vi "runtest Print Selected Reports.vi"(0 "Fields":T1[](array[typedef])=[{"ixField"=0, "iSequenceOrder"=0, "sxFieldId"="Serial Number", "sxSequenceId"="", "sDisplayName"="test", "sValue"="", "sUnits"="", "nDataType"=enum."timestamp", "nNextItem"=enum."Reset", "fSystem"=FALSE, "fSystemValue"=FALSE, "fRequired"=FALSE, "fSetAtTest"=FALSE, "fTestField"=FALSE, "fDeleted"=FALSE, "fIndexed"=FALSE, "fFreeList"=FALSE}, {"ixField"=0, "iSequenceOrder"=0, "sxFieldId"="Model Number", "sxSequenceId"="", "sDisplayName"="test", "sValue"="", "sUnits"="", "nDataType"=enum."timestamp", "nNextItem"=enum."Reset", "fSystem"=FALSE, "fSystemValue"=FALSE, "fRequired"=FALSE, "fSetAtTest"=FALSE, "fTestField"=FALSE, "fDeleted"=FALSE, "fIndexed"=FALSE, "fFreeList"=FALSE}], 1 "sDatasheetsCSV (\"\")":string, 3 "sTestId":string, 5 "Data File Path":path, 9 "Run ID String (\"\")":string, 11 "error in (no error)":errorcluster, 12 "Test Station IP (\"\")":string, 13 "Save Results?":bool, 14 "sxUsername (\"\")":string) -> (15 "error out":errorcluster)   [LabVIEW 2011]
uses:
  server/database/Fields/Field Record.ctl
  server/database/Fields/Field DataTypes.ctl
  server/database/Fields/Field NextItem.ctl
  server/DIAdem/Datasheet/Datasheet Generator Settings.ctl
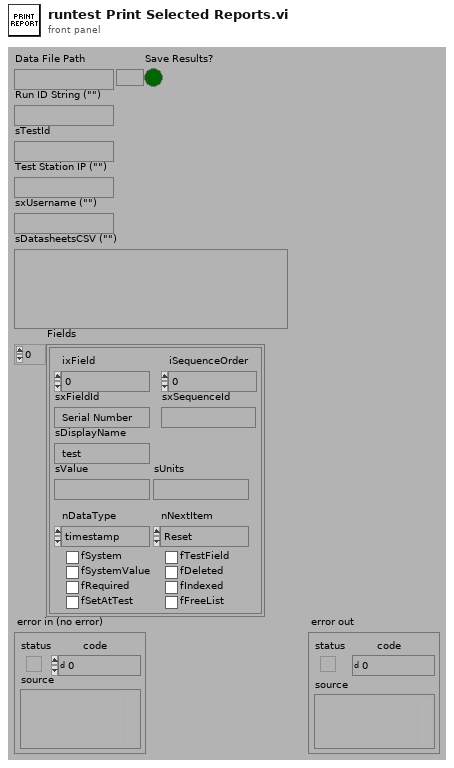
[diagram p1: front panel]
types:
  T1 = typedef "Field Record.ctl" = cluster{"ixField":i32, "iSequenceOrder":i32, "sxFieldId":string, "sxSequenceId":string, "sDisplayName":string, "sValue":string, "sUnits":string, "nDataType":T2, "nNextItem":T3, "fSystem":bool, "fSystemValue":bool, "fRequired":bool, "fSetAtTest":bool, "fTestField":bool, "fDeleted":bool, "fIndexed":bool, "fFreeList":bool}
  T2 = typedef "Field DataTypes.ctl" = enum32{"text", "numeric", "list", "timestamp", "boolean"}
  T3 = typedef "Field NextItem.ctl" = enum32{"Reset", "Retain", "Auto-Increment"}
  T4 = typedef "DATASHEET Generator Settings.ctl" = cluster{"Wait? (t)":bool, "ClientPrint? (f)":bool, "Client (\"\")":string, "joinPDF":bool, "Sort Method":enum16{"Item", "Template", "No Sort"}, "Export Row (-1=all)":i32, "Preview":bool, "Estimate Time":bool, "username":string, "jobid":string}
  T5 = typedef "Connection Refnum.ctl" = cluster{"Environment Handle":i32, "Connection Handle":i32}
  T6 = typedef "TDM_INDEX Record.ctl" = cluster{"Model Number":string, "SN for sort":i32, "Test Type":string, "Test Run":string, "Serial Number":string, "Start Timestamp":timestamp, "Data File":path, "Result Columns":string[]}
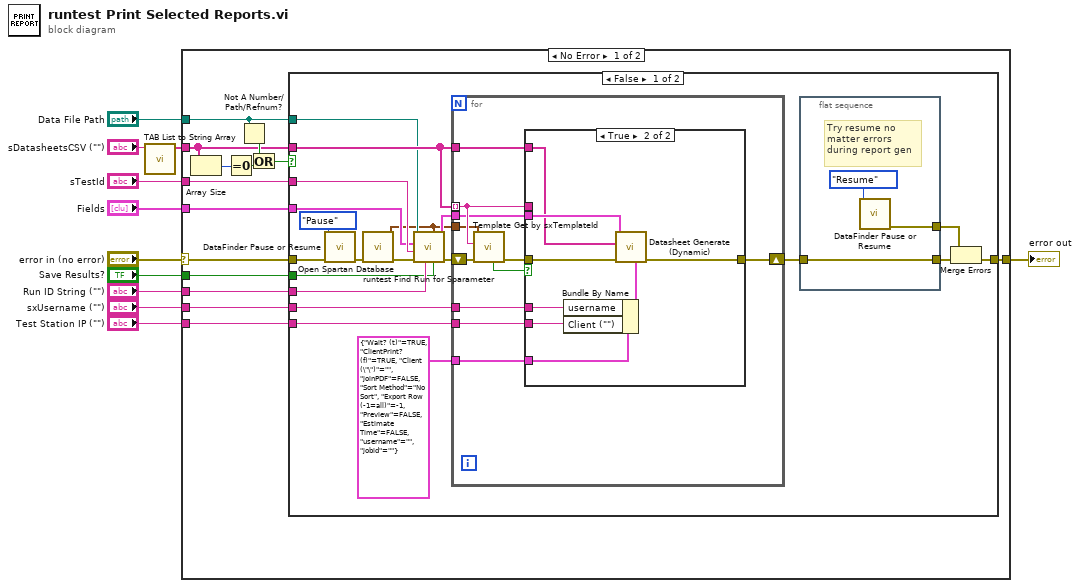
[diagram p0: block diagram]
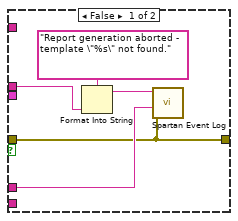
[diagram p2: hidden frame]
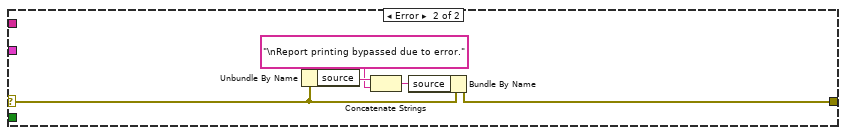
[diagram p4: hidden frame]
diagram:
  n1 = call "TAB List to String Array.vi"("String"="sDatasheetsCSV (\"\")") -> ("Array"=w3:string[])  [unwired: 10 out]
  n2 = case shown="No Error" "error in (no error)" {
    selector: "error in (no error)" -> [w18 w75]
    tunnel: [w21 w74] -> w11
    tunnel: "sxUsername (\"\")" -> [w19 _]
    tunnel: "Run ID String (\"\")" -> [w17 _]
    tunnel: "Data File Path" -> [w12 _]
    tunnel: w3 -> [w15 _]
    tunnel: "Test Station IP (\"\")" -> [w20 _]
    tunnel: "Fields" -> [w16 _]
    tunnel: "sTestId" -> [w14 _]
    tunnel: "Save Results?" -> [w13 _]
    frame No Error {
      n3 = Array Size(array=w15) -> (size(s)=w25:i32)
      n4 = Equal To 0?(x=w25) -> (x = 0?=w23:bool)
      n5 = Not A Number/Path/Refnum?(number/path/refnum=w12) -> (NaN/Path/Refnum?=w24:bool)
      n6 = Or(x=w24, y=w23) -> (x .or. y?=w22:bool)
      n7 = case shown="False" w22 {
        tunnel: w18 -> [w33 w73]
        tunnel: [w28 w73] -> w21
        tunnel: w19 -> [w37 _]
        tunnel: w17 -> [w43 _]
        tunnel: w20 -> [w45 _]
        tunnel: w16 -> [w36 _]
        tunnel: w15 -> [w38 _]
        tunnel: w14 -> [w44 _]
        tunnel: w13 -> [w41 _]
        tunnel: w12 -> [w35 _]
        frame False {
          n8 = call "DataFinder Pause or Resume.vi"("error in (no error)"=w33, "Action"=enum16{"Pause", "Resume"}."Pause") -> ("error out"=w32:errorcluster)  [unwired: 9 in]
          n9 = call "Open Spartan Database.vi"("error in (no error)"=w32) -> ("error out"=w39:errorcluster, "Connection Refnum"=w34:T5)  [unwired: 9 in]
          n10 = call "runtest Find Run for Sparameter.vi"("Save Results?"=w41, "Connection Refnum"=w34, "Run ID"=w43, "error in (no error)"=w39, "Test ID"=w44, "Fields"=w36, "Data File Path"=w35) -> ("error out"=w42:errorcluster, "runs to use"=w40:T6[])  [unwired: 1 in, 2 out]
          n11 = for {
            shift-right: [w58] -> w27
            shift-left: w42 -> [w53]
            tunnel: w37 -> [w59]
            tunnel: w45 -> [w57]
            tunnel: w38 -> [w55] mode=indexing
            tunnel: w40 -> [w54]
            tunnel: w38 -> [w50]
            tunnel: w34 -> [w52]
            tunnel: T4 {"Wait? (t)"=TRUE, "ClientPrint? (f)"=TRUE, "Client (\"\")"="", "joinPDF"=FALSE, "Sort Method"=enum."No Sort", "Export Row (-1=all)"=-1, "Preview"=FALSE, "Estimate Time"=FALSE, "username"="", "jobid"=""} ("Generator Settings") -> [w49]
            n12 = call "Template Get by sxTemplateId.vi"("error in (no error)"=w53, "sxTemplateId (\"\")"=w55, "Connection Refnum"=w52) -> ("error out"=w51:errorcluster, "Data Present"=w56:bool)  [unwired: 7 out]
            n13 = case shown="True" w56 {
              tunnel: w59 -> [w64 w71]
              tunnel: [w61 w69] -> w58
              tunnel: w57 -> [_ w72]
              tunnel: w51 -> [w61 w70]
              tunnel: w55 -> [w63 _]
              tunnel: w54 -> [_ w68]
              tunnel: w50 -> [_ w67]
              tunnel: w49 -> [_ w65]
              frame False {
                n14 = Format Into String(format string="Report generation aborted -  template \"%s\" not found." ("name (unnamed)"), w63) -> (resulting string=w62:string)  [unwired: 2 in, 1 out]
                n15 = call "Spartan Event Log.vi"("error in (no error)"=w61, "username (\"\")"=w64, "message (\"\")"=w62) -> ()  [unwired: 5 in, 1 out]
              }
              frame True {
                n16 = Bundle By Name(cluster=w65, "username"=w71, "Client (\"\")"=w72) -> (w66:T4)
                n17 = call "Datasheet Generate (Dynamic).vi"("Generator Settings"=w66, "error in (no error)"=w70, "Templates"=w67, "Items"=w68) -> ("error out"=w69:errorcluster)  [unwired: 5 in, 2 out]
              }
            }
          }
          n18 = flat-sequence {
            tunnel: [w47] -> w30
            tunnel: w27 -> [w46]
            tunnel: [w46] -> w26
            frame #0 {
              # "Try resume no\nmatter errors\nduring report gen"
              n19 = call "DataFinder Pause or Resume.vi"("Action"=enum16{"Pause", "Resume"}."Resume") -> ("error out"=w47:errorcluster)  [unwired: 10 in]
            }
          }
          n20 = Merge Errors(w30, w26) -> (w28:errorcluster)
        }
        frame True {
        }
      }
    }
    frame Error {
      n21 = Unbundle By Name(w75) -> ("source"=w78:string)
      n22 = Concatenate Strings(w78, "\nReport printing bypassed due to error.") -> (w76:string)
      n23 = Bundle By Name(cluster=w75, "source"=w76) -> (w74:errorcluster)
    }
  }
  "error out" <- w11
